vi "MD420.vi"(0 "MD420.lvclass":refnum<class "MD420.lvclass">, 2 "Temperature Loops":T1 {"3 JEC20 CT001A XQ01" format="%#_13g"}, 3 "Analog Signals from turbine":T2, 4 "From Turbine":T3, 5 "error in":errorcluster) -> (13 "ACT SP Ctrl OFF":bool, 14 "MD420.lvclass out":refnum<class "MD420.lvclass">, 16 "PG Eff SP":dbl, 17 "ACT Eff SP":dbl, 18 "MS Min SP Corr":dbl, 19 "error out":errorcluster)   [LabVIEW 2022 SP3, in "MD420.lvclass"]
uses:
  MD420.lvclass
  MD420.lvclass/MD420.ctl
  SI_modules/SI656/SI656.lvclass
  SI_modules/SI657/SI657.lvclass
  SI_modules/SI101/SI101.lvclass
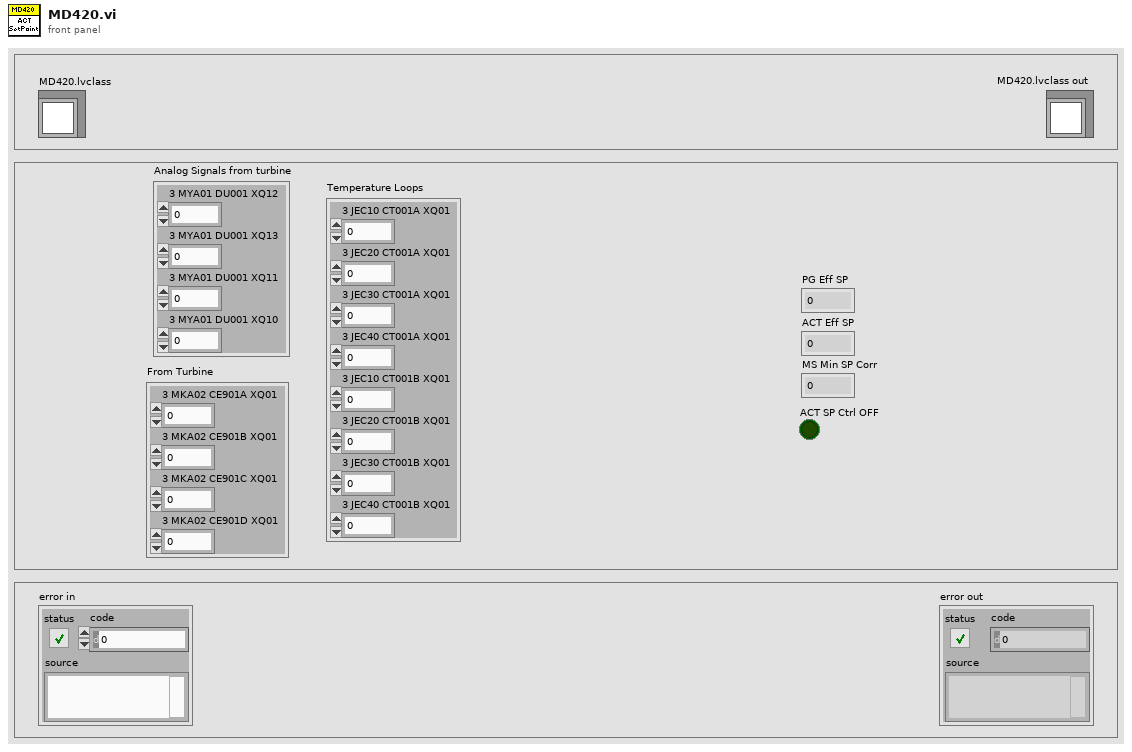
[diagram p1: front panel]
types:
  T1 = cluster{"3 JEC10 CT001A XQ01":dbl, "3 JEC20 CT001A XQ01":dbl, "3 JEC30 CT001A XQ01":dbl, "3 JEC40 CT001A XQ01":dbl, "3 JEC10 CT001B XQ01":dbl, "3 JEC20 CT001B XQ01":dbl, "3 JEC30 CT001B XQ01":dbl, "3 JEC40 CT001B XQ01":dbl}
  T2 = cluster{"3 MYA01 DU001 XQ12":dbl, "3 MYA01 DU001 XQ13":dbl, "3 MYA01 DU001 XQ11":dbl, "3 MYA01 DU001 XQ10":dbl}
  T3 = cluster{"3 MKA02 CE901A XQ01":dbl, "3 MKA02 CE901B XQ01":dbl, "3 MKA02 CE901C XQ01":dbl, "3 MKA02 CE901D XQ01":dbl}
  T4 = cluster{"SUM Ps":dbl, "PG target Setpoint":dbl, "PG < 10%":bool, "PG Setpoint Min":dbl, "PUMA 1/4":bool, "static ACT Setpoint":dbl, "ACT matching value":dbl, "ACT target value":dbl, "ACT 2nd Max":dbl}
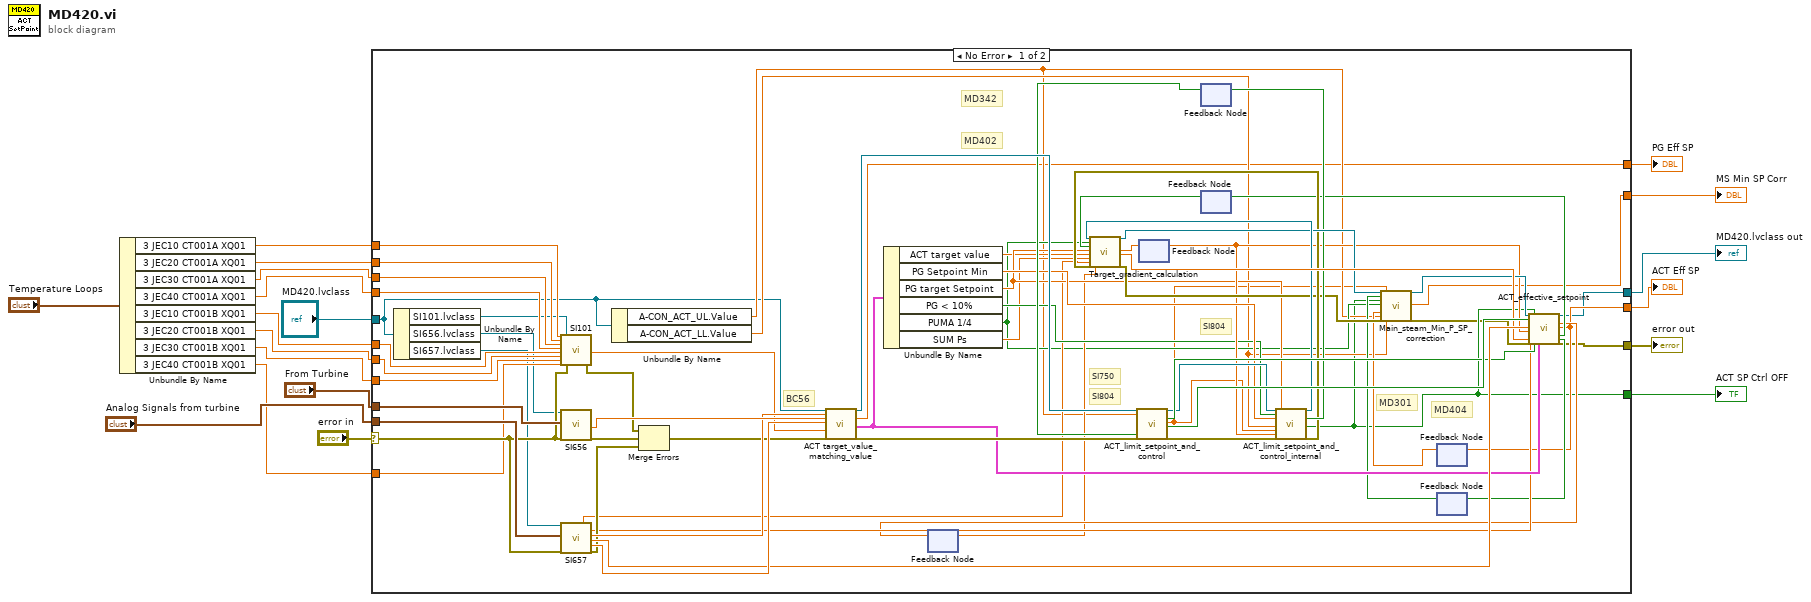
[diagram p0: block diagram]
diagram:
  n1 = Unbundle By Name("Temperature Loops") -> ("3 JEC10 CT001A XQ01"=w8:dbl, "3 JEC20 CT001A XQ01"=w7:dbl, "3 JEC30 CT001A XQ01"=w6:dbl, "3 JEC40 CT001A XQ01"=w5:dbl, "3 JEC10 CT001B XQ01"=w4:dbl, "3 JEC20 CT001B XQ01"=w3:dbl, "3 JEC30 CT001B XQ01"=w2:dbl, "3 JEC40 CT001B XQ01"=w1:dbl)
  n2 = case shown="No Error" "error in" {
    selector: "error in" -> [w77 w85]
    tunnel: "MD420.lvclass" -> [w23 w86]
    tunnel: "From Turbine" -> [w84 _]
    tunnel: "Analog Signals from turbine" -> [w83 _]
    tunnel: [w38 _] -> w15
    tunnel: [w37 _] -> w14
    tunnel: [w36 _] -> w13
    tunnel: [w35 _] -> w12
    tunnel: [w33 w86] -> w11
    tunnel: [w32 w85] -> w10
    tunnel: w8 -> [w31 _]
    tunnel: w7 -> [w30 _]
    tunnel: w6 -> [w29 _]
    tunnel: w5 -> [w28 _]
    tunnel: w4 -> [w27 _]
    tunnel: w3 -> [w26 _]
    tunnel: w2 -> [w25 _]
    tunnel: w1 -> [w24 _]
    frame No Error {
      # "MD301"
      # "SI804"
      # "MD402"
      # "MD342"
      # "SI804"
      # "SI750"
      # "BC56"
      # "MD404"
      n3 = Unbundle By Name(w23) -> ("SI101.lvclass"=w22:refnum<class "SI101.lvclass">, "SI656.lvclass"=w21:refnum<class "SI656.lvclass">, "SI657.lvclass"=w20:refnum<class "SI657.lvclass">)
      n4 = call "SI101.vi"("3 JEC10 CT001A XQ01"=w31, "3 JEC20 CT001A XQ01"=w30, "3 JEC30 CT001A XQ01"=w29, "3 JEC40 CT001A XQ01"=w28, "3 JEC10 CT001B XQ01"=w27, "3 JEC20 CT001B XQ01"=w26, "3 JEC30 CT001B XQ01"=w25, "3 JEC40 CT001B XQ01"=w24, "SI101_AverageReactorCoolantTemperature.lvclass"=w22, "error in"=w77) -> ("error out"=w76:errorcluster, "ACT 2nd Ctrl"=w79:dbl)  [unwired: 13 in, 3 out]
      n5 = call "SI656.vi"("SI656 in"=w21, "From Turbine"=w84, "error in (no error)"=w77) -> ("PG 2nd Min in %"=w82:dbl, "error out"=w75:errorcluster)  [unwired: 13 in, 2 out]
      n6 = call "SI657.vi"("SI657.lvclass"=w20, "Analog Signals from turbine"=w83, "error in (no error)"=w77) -> ("PG SP-Grad"=w49:dbl, "PG eff SP"=w81:dbl, "Switch Ps-Ps_d"=w78:dbl, "PG target SP"=w80:dbl, "error out"=w74:errorcluster)  [unwired: 10 in, 2 out]
      n7 = Unbundle By Name(w23) -> ("A-CON_ACT_UL.Value"=w40:dbl, "A-CON_ACT_LL.Value"=w41:dbl)
      n8 = Merge Errors(w76, w75, w74) -> (w73:errorcluster)
      n9 = call "ACT target_value_matching_value.vi"("MD420.lvclass"=w23, "PG eff SP"=w81, "PG 2nd Min in %"=w82, "PG target SP"=w80, "ACT 2nd Ctrl"=w79, "error in (no error)"=w73) -> ("MD420.lvclass out"=w69:refnum<class "MD420.lvclass">, "PG Eff SP"=w38:dbl, "Internal Outputs"=w58:T4, "error out"=w62:errorcluster)  [unwired: 18 in]
      n10 = Unbundle By Name(w58) -> ("ACT target value"=w48:dbl, "PG Setpoint Min"=w57:dbl, "PG target Setpoint"=w53:dbl, "PG < 10%"=w54:bool, "PUMA 1/4"=w43:bool, "SUM Ps"=w52:dbl)
      n11 = feedback #1() -> (w46:dbl)  [unwired: 1 in]
      n12 = feedback #2() -> (w55:dbl)  [unwired: 1 in]
      n13 = feedback #3() -> (w63:bool)  [unwired: 1 in]
      n14 = call "ACT_limit_setpoint_and_control.vi"("MD420.lvclass in"=w69, "ACT upper limit"=w40, "Increase ACT limit Setpoint"=w63, "error out"=w62) -> ("MD420.lvclass out"=w68:refnum<class "MD420.lvclass">, "Release +0,6 K/min"=w71:bool, "ACT limit Setpoint"=w39:dbl, "ACT limit Setpoint\ndecreased"=w72:bool, "error out"=w61:errorcluster)  [unwired: 19 in]
      n15 = feedback #4() -> (w50:bool)  [unwired: 1 in]
      n16 = call "ACT_limit_setpoint_and_control_internal.vi"("MD420.lvclass"=w68, "PG < 10%"=w54, "PG Setpoint Min"=w57, "ACT lower limit"=w41, "ACT limit Setpoint"=w39, "PG1"=w55, "error in"=w61, "PG target Setpoint"=w53) -> ("MD420.lvclass out"=w67:refnum<class "MD420.lvclass">, "Increase ACT\nlimit Setpoint"=w64:bool, "ACT SP Ctrl\nOFF"=w36:bool, "error out"=w60:errorcluster)  [unwired: 16 in]
      n17 = call "Target_gradient_calculation.vi"("MD420.lvclass"=w67, "PUMA 1/4"=w43, "Load change"=w50, "PG target Setpoint"=w53, "ACT target value"=w48, "SUM Ps"=w52, "Ps Grad"=w49, "error in"=w60, "ACT Eff SP (k-1)"=w46) -> ("MD420.lvclass out"=w66:refnum<class "MD420.lvclass">, "PG1"=w56:dbl, "Target Grad"=w70:dbl, "error out"=w59:errorcluster)  [unwired: 15 in]
      n18 = feedback-in #2(w56) -> ()
      n19 = feedback-in #3(w64) -> ()
      n20 = feedback #5() -> (w42:dbl)  [unwired: 1 in]
      n21 = feedback #6() -> (w44:bool)  [unwired: 1 in]
      n22 = call "Main_steam_Min_P_SP_correction.vi"("MD420.lvclass in"=w66, "Min-P Corr OFF"=w44, "ACT SP Ctrl OFF"=w36, "PUMA 1/4"=w43, "ACT effective Setpoint"=w42, "ACT upper limit"=w40, "error in"=w59, "ACT limit Setpoint"=w39, "ACT lower limit"=w41) -> ("MD420.lvclass out"=w65:refnum<class "MD420.lvclass">, "MS Min SP Corr"=w35:dbl, "error out"=w34:errorcluster)  [unwired: 16 in]
      n23 = call "ACT_effective_setpoint.vi"("MD420.lvclass"=w65, "ACT limit Setpoint decreased"=w72, "Switch Ps-Ps_d (SI657)"=w78, "PG1"=w55, "PG SP-Grad(SI657)"=w49, "Target Grad"=w70, "error in (no error)"=w34, "ACT-Ctrl OFF (MD404)"=w36, "Release +0,6 K/min"=w71, "Internal Outputs"=w58) -> ("MD420.lvclass out"=w33:refnum<class "MD420.lvclass">, "ACT Eff SP k-1"=w47:dbl, "ACT Eff SP"=w37:dbl, "Load Change"=w51:bool, "Min-P Corr OFF"=w45:bool, "error out"=w32:errorcluster)  [unwired: 11 in, 1 out]
      n24 = feedback-in #1(w47) -> ()
      n25 = feedback-in #4(w51) -> ()
      n26 = feedback-in #5(w37) -> ()
      n27 = feedback-in #6(w45) -> ()
    }
    frame Error {
    }
  }
  "PG Eff SP" <- w15
  "ACT Eff SP" <- w14
  "ACT SP Ctrl OFF" <- w13
  "MS Min SP Corr" <- w12
  "MD420.lvclass out" <- w11
  "error out" <- w10
